vi "Play Sound.vi"(8 "error in (no error)":errorcluster, 11 "Application In":refnum<class "Application.lvclass">=refnum) -> (0 "error out":errorcluster)   [LabVIEW 2021]
uses:
  <vilib>/sound2/lvsound2.llb/Sound Output Task ID.ctl
  LVApp/Modules/Sound Manager/Typedefs/Sound Effects.ctl
  Application/Application.lvclass
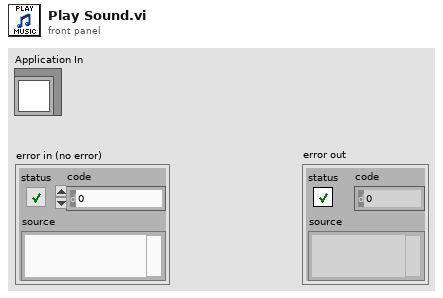
[diagram p1: front panel]
types:
  T1 = typedef "Sound Effects.ctl" = enum16{"Bomb In", "Bomb Out", "Bomb Touched", "Game Over", "Victory", "Eat", "10 Fruits", "Eat2", "Eat3", "Eat4", "MaxShield", "Shield", "10p", "Grape In", "Grape Out", "20p", "30p", "40p", "50p", "60p", "70p", "80p", "90p", "100p", "All shields cracked", "Mouse In", "Mouse Out", "Mouse Eaten", "Grape Eaten", "States Recover", "Broken Shield", "Bonus", "Happy Time", "explode", "Game over musica", "Back Music", "Shield Catch", "Evil lough", "Cricket In", "Cricket eaten", "Lets Go", "Jump1", "Jump2", "Jump3", "Unstoppable", "Troll Music", "winner"}
  T2 = typedef "Sound Output Task ID.ctl" = u32
  T3 = cluster{"Sound Effect":T1, "Task ID":T2, "Init":timestamp}[]
  T4 = typedef "Application.lvclass/Sound Effects.ctl" = enum16{"Bomb In", "Bomb Out", "Bomb Touched", "Game Over", "Victory", "Eat", "10 Fruits", "Eat2", "Eat3", "Eat4", "MaxShield", "Shield", "10p", "Grape In", "Grape Out", "20p", "30p", "40p", "50p", "60p", "70p", "80p", "90p", "100p", "All shields cracked", "Mouse In", "Mouse Out", "Mouse Eaten", "Grape Eaten", "States Recover", "Broken Shield", "Bonus", "Happy Time", "explode", "Game over musica", "Back Music", "Shield Catch", "Evil lough", "Cricket In", "Cricket eaten", "Lets Go", "Jump1", "Jump2", "Jump3", "Unstoppable", "Troll Music", "winner"}
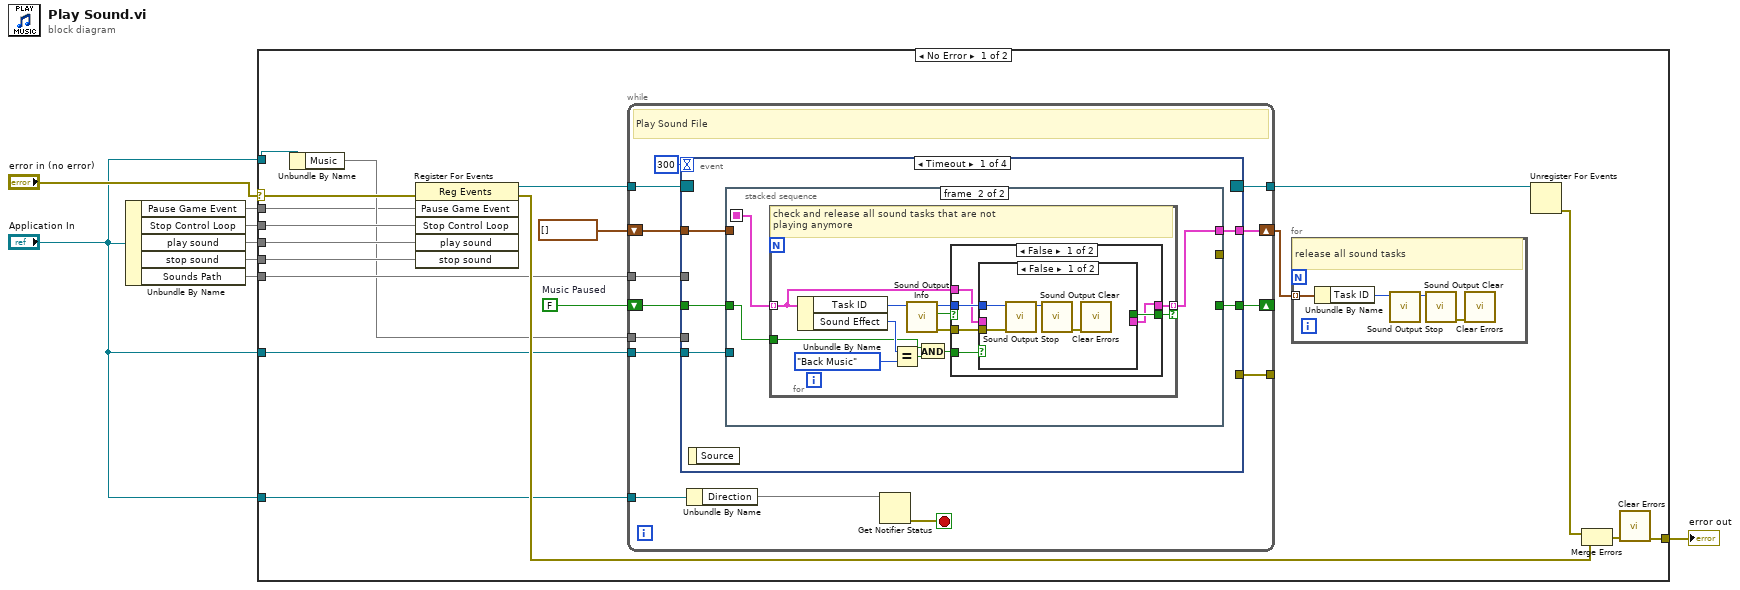
[diagram p0: block diagram]
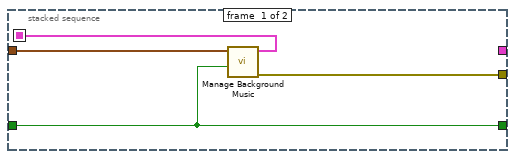
[diagram p2: hidden frame]
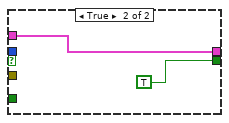
[diagram p4: hidden frame]
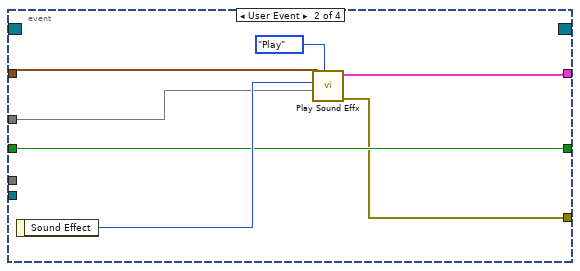
[diagram p5: hidden frame]
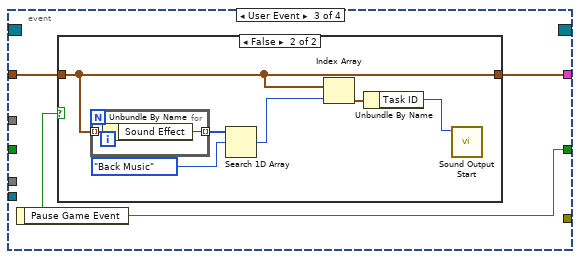
[diagram p6: hidden frame]
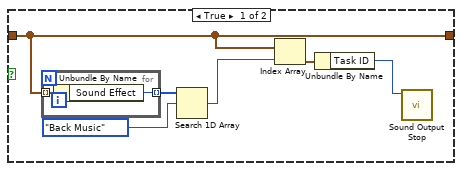
[diagram p7: hidden frame]
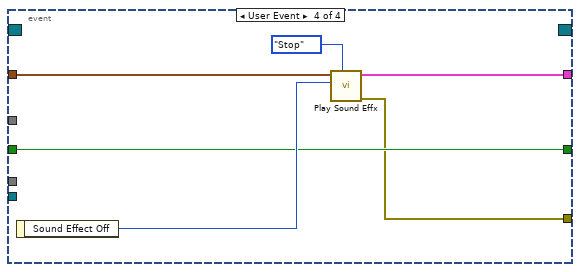
[diagram p8: hidden frame]
diagram:
  n1 = Unbundle By Name("Application In") -> ("Pause Game Event"=w1, "Stop Control Loop"=w6, "play sound"=w5, "stop sound"=w4, "Sounds Path"=w3)
  n2 = case shown="No Error" "error in (no error)" {
    selector: "error in (no error)" -> [w22 w116]
    tunnel: w6 -> [w21 _]
    tunnel: [w23 w116] -> w8
    tunnel: "Application In" -> [w14 _]
    tunnel: w5 -> [w19 _]
    tunnel: w4 -> [w15 _]
    tunnel: w3 -> [w16 _]
    tunnel: "Application In" -> [w12 _]
    tunnel: "Application In" -> [w11 _]
    tunnel: w1 -> [w9 _]
    frame No Error {
      w10 = FALSE  # Music Paused
      n3 = Unbundle By Name(w14) -> ("Music"=w13)
      n4 = register-events(error in=w22, w9, w21, w19, w15) -> (reference out=w18:refnum<event-registration>, error out=w25:errorcluster)  [unwired: 1 in]
      n5 = while {
        tunnel: w18 -> [w40]
        tunnel: [w39] -> w27
        shift-right: [w36] -> w20
        shift-left: cluster{"Sound Effect":T1, "Task ID":T2}[] [] -> [w38]
        tunnel: w16 -> [w37]
        tunnel: w13 -> [w35]
        tunnel: w12 -> [w34]
        tunnel: w11 -> [w32]
        shift-right: [w29] -> _
        shift-left: w10 -> [w30]
        tunnel: [w28] -> _
        stop <- w31 stop-if-true
        # "Play Sound File"
        n6 = event shown="[0] Timeout" {
          selector: w40 -> [_ _ _ _]
          dyn-events: [_ _ _ _] -> w39
          timeout: 300 -> [_ _ _ _]
          tunnel: w38 -> [w46 w85 w89 w110]
          tunnel: [w45 w84 w88 w109] -> w36
          tunnel: w37 -> [_ w82 _ _]
          tunnel: w35 -> [_ _ _ _]
          tunnel: w34 -> [w44 _ _ _]
          tunnel: w30 -> [w43 w81 _ w108]
          tunnel: [w42 w81 w87 w108] -> w29
          tunnel: [_ w80 _ w106] -> w28
          event Timeout {
            n7 = event-data() -> ()  [unwired: 1 in, 1 out]
            n8 = stacked-sequence {
              seq-local: [w49 _] -> [_ w52]
              tunnel: w46 -> [w50 _]
              tunnel: [_ w53] -> w45
              tunnel: w44 -> [_ _]
              tunnel: w43 -> [w48 w51]
              tunnel: [w48 _] -> w42
              tunnel: [w47 _] -> _
              frame #0 {
                n9 = call "Manage Background Music.vi"("Music Paused"=w48, "Sounds"=w50) -> ("error out"=w47:errorcluster, "Sounds Out"=w49:T3)  [unwired: 7 in, 1 out]
              }
              frame #1 {
                n10 = for {
                  tunnel: w52 -> [w59] mode=indexing
                  tunnel: [w62] -> w53 mode=indexing if=w61
                  tunnel: w51 -> [w54]
                  # "check and release all sound tasks that are not \nplaying anymore"
                  n11 = Unbundle By Name(w59) -> ("Task ID"=w60:T2, "Sound Effect"=w58:T1)
                  n12 = Equal?(x=w58, y=Sound_Effects."Back Music") -> (x = y?=w56:bool)
                  n13 = call <vilib>:"Sound Output Info.vi"("task ID"=w60) -> ("error out"=w64:errorcluster, "is playing?"=w65:bool, "task ID out"=w63:T2)  [unwired: 7 in, 1 out]
                  n14 = And(x=w54, y=w56) -> (x .and. y?=w55:bool)
                  n15 = case shown="False" w65 {
                    tunnel: w64 -> [w71 _]
                    tunnel: w63 -> [w70 _]
                    tunnel: [w66 w78] -> w62
                    tunnel: [w68 TRUE] -> w61
                    tunnel: w59 -> [w67 w78]
                    tunnel: w55 -> [w69 _]
                    frame False {
                      n16 = case shown="False" w69 {
                        selector: w69 -> [_ w77]
                        tunnel: w71 -> [w73 _]
                        tunnel: w70 -> [w72 _]
                        tunnel: [_ w77] -> w68
                        tunnel: w67 -> [_ w76]
                        tunnel: [_ w76] -> w66
                        frame False {
                          n17 = call <vilib>:"Sound Output Stop.vi"("error in (no error)"=w73, "task ID"=w72) -> ("task ID out"=w74:T2)  [unwired: 8 in, 1 out]
                          n18 = call <vilib>:"Sound Output Clear.vi"("task ID"=w74) -> ("error out"=w75:errorcluster)  [unwired: 10 in]
                          n19 = call <vilib>:"Clear Errors.vi"("error in (no error)"=w75) -> ()  [unwired: 5 in, 2 out]
                        }
                        frame True {
                          # "back music and paused, \ndo not clear"
                        }
                      }
                    }
                    frame True {
                    }
                  }
                }
              }
            }
          }
          event User Event {
            n20 = event-data() -> ("Sound Effect"=w83:T4)  [unwired: 1 in]
            n21 = call "Play Sound Effx.vi"("event"=enum16{"Play", "Stop"}."Play", "path"=w82, "Sound Effect Off"=w83, "Sounds In"=w85) -> ("error out"=w80:errorcluster, "Sounds Out"=w84:T3)  [unwired: 6 in]
          }
          event User Event {
            n22 = event-data() -> ("Pause Game Event"=w87:bool)  [unwired: 1 in]
            n23 = case shown="False" w87 {
              tunnel: w89 -> [w91 w99]
              tunnel: [w91 w99] -> w88
              frame True {
                n24 = for {
                  tunnel: w91 -> [w97] mode=indexing
                  tunnel: [w96] -> w93 mode=indexing
                  n25 = Unbundle By Name(w97) -> ("Sound Effect"=w96:T1)
                }
                n26 = Search 1D Array(1D array=w93, element=Sound_Effects."Back Music") -> (index of element=w92:i32)  [unwired: 1 in]
                n27 = Index Array(array=w91, index=w92) -> (element=w95:cluster{"Sound Effect":T1, "Task ID":T2})
                n28 = Unbundle By Name(w95) -> ("Task ID"=w90:T2)
                n29 = call <vilib>:"Sound Output Stop.vi"("task ID"=w90) -> ()  [unwired: 9 in, 2 out]
              }
              frame False {
                n30 = for {
                  tunnel: w99 -> [w105] mode=indexing
                  tunnel: [w104] -> w101 mode=indexing
                  n31 = Unbundle By Name(w105) -> ("Sound Effect"=w104:T1)
                }
                n32 = Search 1D Array(1D array=w101, element=Sound_Effects."Back Music") -> (index of element=w100:i32)  [unwired: 1 in]
                n33 = Index Array(array=w99, index=w100) -> (element=w103:cluster{"Sound Effect":T1, "Task ID":T2})
                n34 = Unbundle By Name(w103) -> ("Task ID"=w98:T2)
                n35 = call <vilib>:"Sound Output Start.vi"("task ID"=w98) -> ()  [unwired: 9 in, 2 out]
              }
            }
          }
          event User Event {
            n36 = event-data() -> ("Sound Effect Off"=w111:T4)  [unwired: 1 in]
            n37 = call "Play Sound Effx.vi"("event"=enum16{"Play", "Stop"}."Stop", "Sound Effect Off"=w111, "Sounds In"=w110) -> ("error out"=w106:errorcluster, "Sounds Out"=w109:T3)  [unwired: 7 in]
          }
        }
        n38 = Unbundle By Name(w32) -> ("Direction"=w33)
        n39 = Get Notifier Status(notifier=w33) -> (error out=w31:errorcluster)  [unwired: 1 in, 4 out]
      }
      n40 = for {
        tunnel: w20 -> [w113] mode=indexing
        # "release all sound tasks"
        n41 = Unbundle By Name(w113) -> ("Task ID"=w112:T2)
        n42 = call <vilib>:"Sound Output Stop.vi"("task ID"=w112) -> ("task ID out"=w114:T2)  [unwired: 9 in, 1 out]
        n43 = call <vilib>:"Sound Output Clear.vi"("task ID"=w114) -> ("error out"=w115:errorcluster)  [unwired: 10 in]
        n44 = call <vilib>:"Clear Errors.vi"("error in (no error)"=w115) -> ()  [unwired: 5 in, 2 out]
      }
      n45 = Unregister For Events(event registration refnum=w27) -> (error out=w26:errorcluster)  [unwired: 1 in]
      n46 = Merge Errors(w26, w25) -> (w24:errorcluster)
      n47 = call <vilib>:"Clear Errors.vi"("error in (no error)"=w24) -> ("error out"=w23:errorcluster)  [unwired: 5 in, 1 out]
    }
    frame Error {
    }
  }
  "error out" <- w8
